vi "Apply.vi"(8 "Error In":errorcluster, 11 "HAL:HDO4000A Base CFG in":refnum<class "HDO4000A Base CFG.lvclass">) -> (0 "Error Out":errorcluster, 3 "HAL:HDO4000A Base CFG out":refnum<class "HDO4000A Base CFG.lvclass">)   [LabVIEW 2023]
uses:
  HDO4000A Base CFG.lvclass
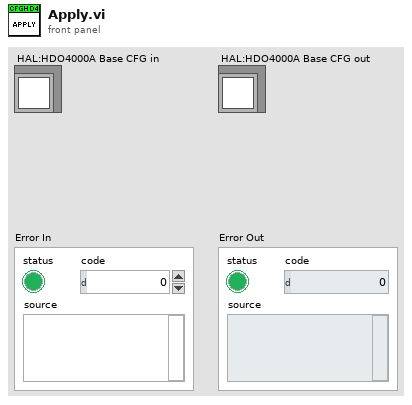
[diagram p1: front panel]
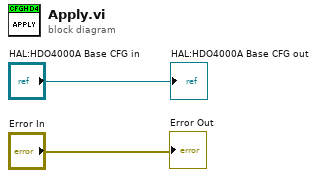
[diagram p0: block diagram]
diagram:
  "Error Out" <- "Error In"
  "HAL:HDO4000A Base CFG out" <- "HAL:HDO4000A Base CFG in"
